vi "Write Value.vi"(7 "GPIO":refnum<class "GPIO.lvclass">, 8 "error in (no error)":errorcluster, 10 "Value":bool, 11 "Session In":refnum<class "Session.lvclass">) -> (0 "error out":errorcluster, 3 "Session Out":refnum<class "Session.lvclass">)   [LabVIEW 2024, in "CTI.lvlib" / "GPIO.lvclass"]
uses:
  GPIO.lvclass
  Session/Session.lvclass
  GPIO.lvclass/GPIO.ctl
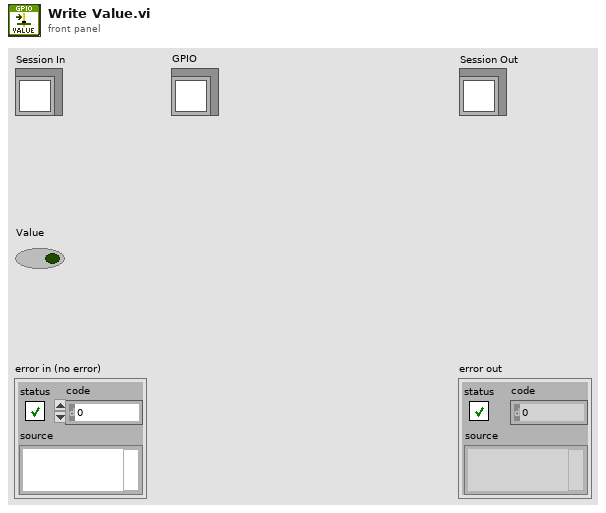
[diagram p1: front panel]
types:
  T1 = typedef "CTI.lvlib/GPIO Number.ctl" = i8
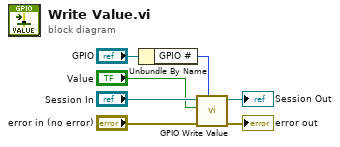
[diagram p0: block diagram]
diagram:
  n1 = Unbundle By Name("GPIO") -> ("GPIO #"=w4:T1)
  n2 = call "GPIO Write Value.vi"("GPIO #"=w4, "error in (no error)"="error in (no error)", "Value"="Value", "Session in"="Session In") -> ("error out"=→"error out":errorcluster, "Session out"=→"Session Out":refnum<class "Session.lvclass">)  [unwired: 6 in]
